vi "TDMS(Create).vi"(8 "error in (no error)":errorcluster caption="错误输入（无错误）", 11 "文件名":string) -> (0 "error out":errorcluster caption="错误输出", 3 "tdms file out":refnum<k34>)   [LabVIEW 2020, in "人体健康监测系统.lvclass"]
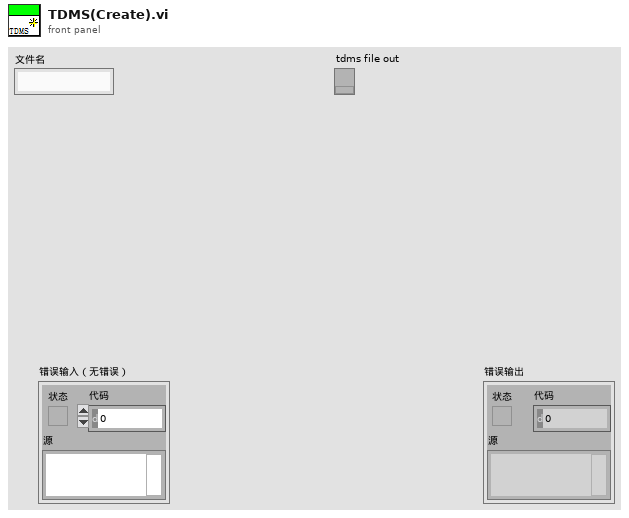
[diagram p1: front panel]
types:
  T1 = enum16{"open", "open or create", "create or replace", "create", "open (read-only)"}
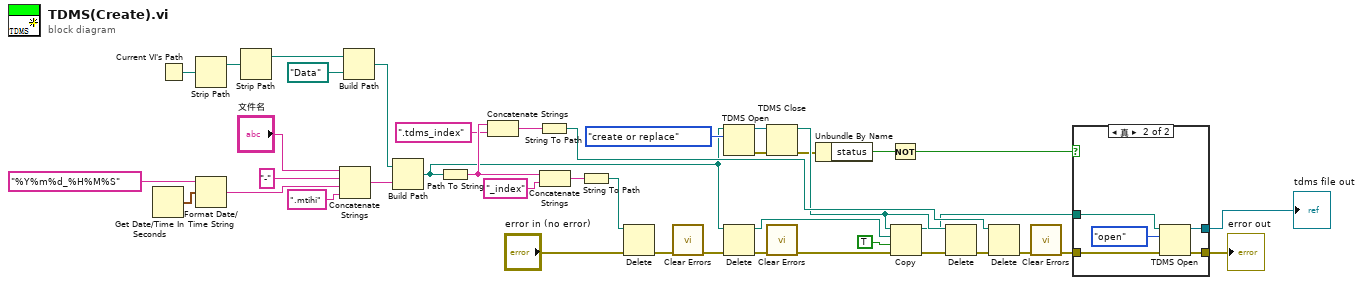
[diagram p0: block diagram]
diagram:
  n1 = Get Date/Time In Seconds() -> (seconds since 1Jan1904=w20:timestamp)
  n2 = Current VI's Path() -> (path=w9:path)
  n3 = Strip Path(path=w9) -> (stripped path=w8:path)  [unwired: 1 out]
  n4 = Format Date/Time String(time format string (%c)="%Y%m%d_%H%M%S" ("时间格式字符串(%c)"), seconds (now)=w20) -> (date/time string=w17:string)  [unwired: 1 in]
  n5 = Strip Path(path=w8) -> (stripped path=w7:path)  [unwired: 1 out]
  n6 = Concatenate Strings("文件名", "-" ("字符串"), w17, ".mtihi" ("字符串")) -> (w15:string)
  n7 = Build Path(base path=w7, name or relative path=path "Data" ("名称或相对路径")) -> (appended path=w5:path)
  n8 = Build Path(base path=w5, name or relative path=w15) -> (appended path=w14:path)
  n9 = Path To String(path=w14) -> (string=w39:string)
  n10 = Concatenate Strings(w39, ".tdms_index" ("字符串")) -> (w30:string)
  n11 = String To Path(string=w30) -> (path=w31:path)
  n12 = Concatenate Strings(w39, "_index" ("字符串")) -> (w37:string)
  n13 = String To Path(string=w37) -> (path=w36:path)
  n14 = Delete(path (use dialog)=w36, error in="error in (no error)") -> (error out=w40:errorcluster)  [unwired: 3 in, 2 out]
  n15 = call <vilib>:"Clear Errors.vi"("error in (no error)"=w40) -> ("error out"=w41:errorcluster)  [unwired: 5 in, 1 out]
  n16 = TDMS Open(10:T1."create or replace" ("操作(0:open)"), 11:w14) -> (0:w23:errorcluster, 3:w24:refnum<k34>)  [unwired: 5 in]
  n17 = Delete(path (use dialog)=w14, error in=w41) -> (deleted path=w33:path, error out=w34:errorcluster)  [unwired: 3 in, 1 out]
  n18 = TDMS Close(8:w23, 11:w24) -> (0:w11:errorcluster, 3:w26:path)
  n19 = call <vilib>:"Clear Errors.vi"("error in (no error)"=w34) -> ("error out"=w35:errorcluster)  [unwired: 5 in, 1 out]
  n20 = Unbundle By Name(w11) -> ("status"=w22:bool)
  n21 = Not(x=w22) -> (.not. x?=w10:bool)
  n22 = Copy(8:w35, 9:TRUE ("覆盖(F)"), 10:w33, 11:w26) -> (0:w27:errorcluster, 3:w12:path)  [unwired: 1 in, 1 out]
  n23 = Delete(path (use dialog)=w26, error in=w27) -> (error out=w32:errorcluster)  [unwired: 3 in, 2 out]
  n24 = Delete(path (use dialog)=w31, error in=w32) -> (error out=w21:errorcluster)  [unwired: 3 in, 2 out]
  n25 = call <vilib>:"Clear Errors.vi"("error in (no error)"=w21) -> ("error out"=w13:errorcluster)  [unwired: 5 in, 1 out]
  n26 = case shown="真" w10 {
    tunnel: w13 -> [w42 w46]
    tunnel: w12 -> [_ w45]
    tunnel: [_ w44] -> w4
    tunnel: [w42 w43] -> w2
    frame False {
    }
    frame True {
      n27 = TDMS Open(8:w46, 10:T1."open" ("操作(0:open)"), 11:w45) -> (0:w43:errorcluster, 3:w44:refnum<k34>)  [unwired: 4 in]
    }
  }
  "error out" <- w2
  "tdms file out" <- w4
